vi "RT Create Target Disk Image.vi"(6 "file blacklist":string[](array[string]), 8 "error in (no error)":errorcluster, 9 "allow overwrite? (F)":bool, 10 "image file path":path, 11 "target address":string) -> (0 "error out":errorcluster, 2 "image file path out":path, 3 "target address out":string)   [LabVIEW 2020, in "NI_Real-Time Libraries.lvlib"]
doc: "LabVIEW no longer supports this VI. For information about replacing the RT Utility VIs, refer to ni.com/info and enter the Info Code RT_Utility_Replace. Copies the contents of the primary hard drive on the RT target to the local zip file you specify using the <B>image file path</B> input.\n\n<B>target address</B> specifies the IP address or DNS name of the target. \n\n<B>image file path</B> specifies the name and location of the RT target disk image on the local computer. To ensure compatibility, National Instruments recommends that you use a file name with a .zip extension. \n\n<B>allow overwrite?</B> specifies whether this VI can overwrite an existing file at the specified <B>image file path</B>. If <B>allow overwrite?</B> is TRUE, this VI overwrites the contents of <B>image file path</B>. If <B>allow overwrite?</B> is FALSE and <B>image file path</B> already exists on the local computer, this VI returns an error. \n\n<B>error in</B> describes error conditions that occur before this node runs. This input provides standard error in functionality. \n\n<B>file blacklist</B> specifies an array of file paths to exclude from the target image. To enable filtering through strict matching, the data type of this control is an array of strings rather than an array of paths. \n\n<B>target address out</B> returns the same address as <B>target address</B>. \n\n<B>image file path out</B> returns the same path as <B>image path</B>. \n\n<B>error out</B> contains error information. This output provides standard error out functionality. \n\n\nRT Create Target Disk Image Details\nThis VI stores the RT target disk image as a ZIP file. Use the RT Apply Target Disk Image VI to apply the disk images you create using this VI. This VI does not support disk images based on RT targets with multiple operating systems or multiple hard disk partitions."
uses:
  <vilib>/real-time/NI_Real-Time Libraries.lvlib
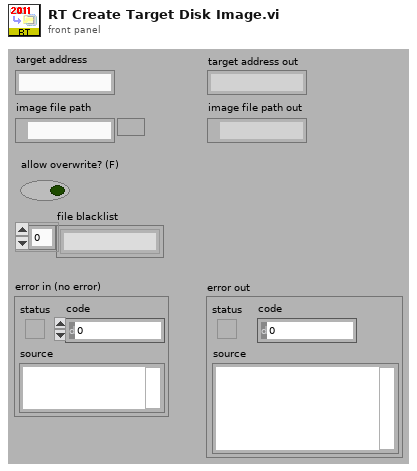
[diagram p1: front panel]
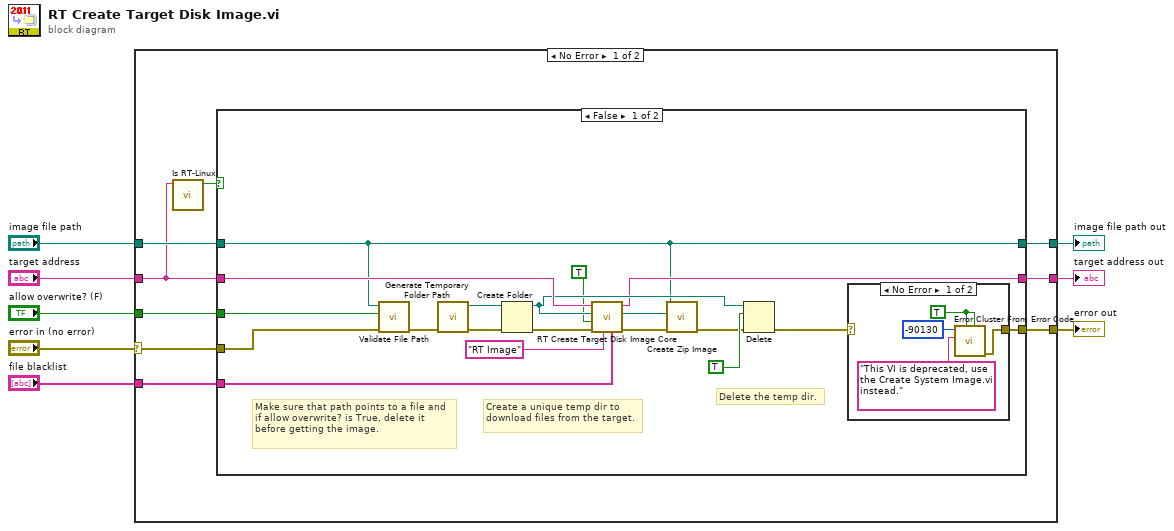
[diagram p0: block diagram]
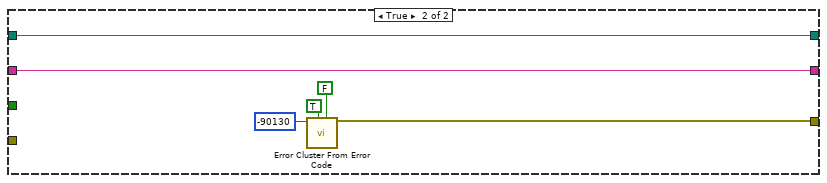
[diagram p3: hidden frame]
diagram:
  n1 = case shown="No Error" "error in (no error)" {
    selector: "error in (no error)" -> [w14 w50]
    tunnel: "target address" -> [w9 w48]
    tunnel: "file blacklist" -> [w16 _]
    tunnel: "allow overwrite? (F)" -> [w15 _]
    tunnel: "image file path" -> [w13 w49]
    tunnel: [w17 w50] -> w3
    tunnel: [w11 w49] -> w2
    tunnel: [w12 w48] -> w1
    frame No Error {
      n2 = call <vilib>:"Is RT-Linux.vi"("target address"=w9) -> ("Is RT-Linux?"=w10:bool)  [unwired: 10 in]
      n3 = case shown="False" w10 {
        tunnel: w9 -> [w36 w46]
        tunnel: [w18 w47] -> w17
        tunnel: w16 -> [w29 _]
        tunnel: w15 -> [w27 _]
        tunnel: w14 -> [w22 _]
        tunnel: w13 -> [w20 w45]
        tunnel: [w21 w46] -> w12
        tunnel: [w20 w45] -> w11
        frame False {
          # "Make sure that path points to a file and if allow overwrite? is True, delete it before getting the image."
          # "Delete the temp dir."
          # "Create a unique temp dir to download files from the target."
          n4 = call <vilib>:"Validate File Path.vi"("error in (no error)"=w22, "allow overwrite (False)?"=w27, "image file path"=w20) -> ("error out"=w26:errorcluster)  [unwired: 8 out]
          n5 = call <vilib>:"Generate Temporary Folder Path.vi"("error in (no error)"=w26) -> ("error out"=w35:errorcluster, "Unique Temporary Folder Path"=w33:path)  [unwired: 9 out]
          n6 = Create Folder(path (use dialog)=w33, error in=w35) -> (created path=w32:path, error out=w34:errorcluster)  [unwired: 1 in, 1 out]
          n7 = call <vilib>:"RT Create Target Disk Image Core.vi"("file blacklist"=w29, "image name"="RT Image", "error in (no error)"=w34, "allow overwrite? (F)"=TRUE ("allow overwrite (False)?"), "base path"=w32, "target address"=w36) -> ("error out"=w23:errorcluster, "image path"=w24:path, "target address out"=w21:string)  [unwired: 3 out]
          n8 = call <vilib>:"Create Zip Image.vi"("error in (no error)"=w23, "image path"=w24, "image file path"=w20) -> ("error out"=w25:errorcluster)  [unwired: 8 out]
          n9 = Delete(path (use dialog)=w32, entire hierarchy (F)=TRUE ("confirm (F)"), error in=w25) -> (error out=w19:errorcluster)  [unwired: 4 out]
          n10 = case shown="No Error" w19 {
            selector: w19 -> [_ w41]
            tunnel: [w37 w41] -> w18
            frame No Error {
              w39 = TRUE ("show call chain? (False)")
              n11 = call <vilib>:"Error Cluster From Error Code.vi"("is warning? (False)"=w39, "show call chain? (False)"=w39, "error message (\"\")"="This VI is deprecated, use the Create System Image.vi instead.", "error code (0)"=-90130) -> ("error out"=w37:errorcluster)  [unwired: 5 in]
            }
            frame Error {
            }
          }
        }
        frame True {
          n12 = call <vilib>:"Error Cluster From Error Code.vi"("is warning? (False)"=FALSE, "show call chain? (False)"=TRUE, "error code (0)"=-90130) -> ("error out"=w47:errorcluster)  [unwired: 6 in]
        }
      }
    }
    frame Error {
    }
  }
  "error out" <- w3
  "image file path out" <- w2
  "target address out" <- w1
